vi "Temperature Warnings.vi"(8 "错误输入":cluster{"状态":bool, "代码":i32, "源":string}, 9 "最低温度":dbl, 10 "最高温度":dbl, 11 "当前温度":dbl) -> (0 "错误输出":cluster{"状态":bool, "代码":i32, "源":string}, 2 "警告文本":string="无警告", 3 "警告？":bool)   [LabVIEW 2012]
doc: "该练习将为子VI创建图标和连线板，然后在调用VI中测试调用子VI。"
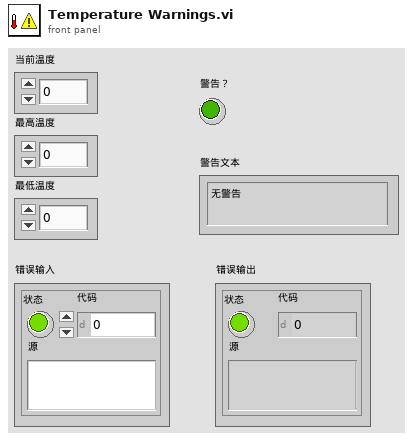
[diagram p1: front panel]
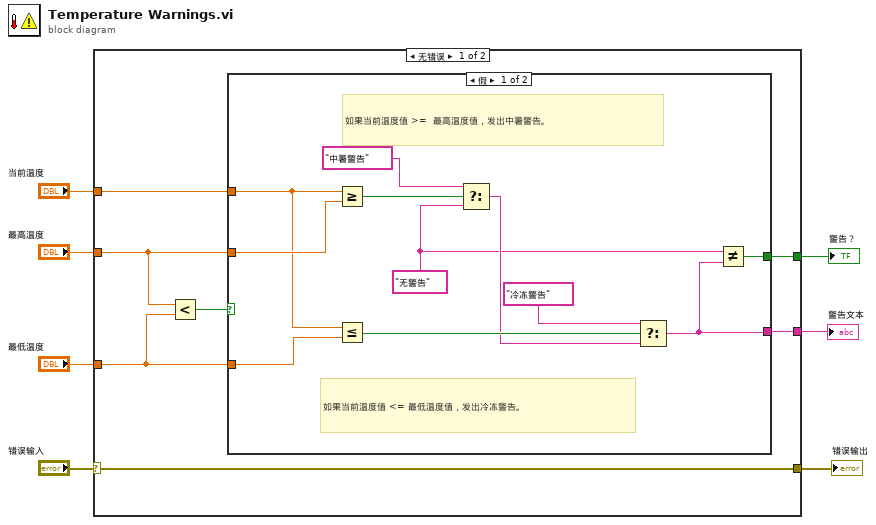
[diagram p0: block diagram]
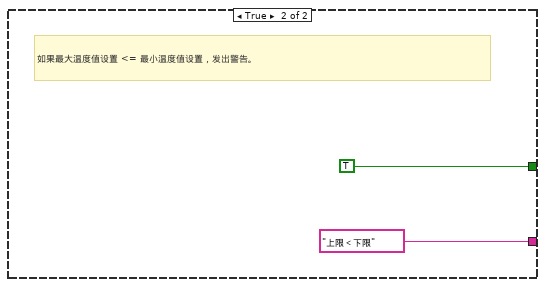
[diagram p2: hidden frame]
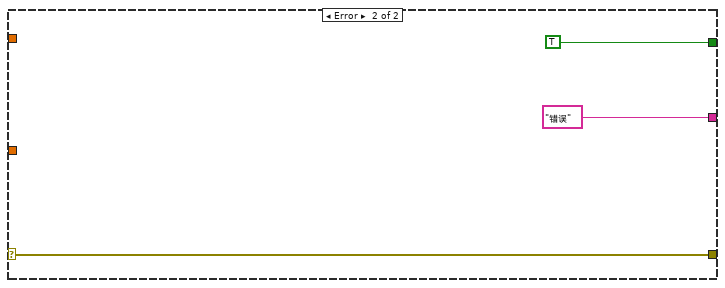
[diagram p3: hidden frame]
diagram:
  n1 = case shown="无错误" "错误输入" {
    selector: "错误输入" -> [w12 w30]
    tunnel: [w14 "错误" ("f")] -> w1
    tunnel: [w13 TRUE] -> w2
    tunnel: [w12 w30] -> w6
    tunnel: "最低温度" -> [w9 _]
    tunnel: "当前温度" -> [w11 _]
    tunnel: "最高温度" -> [w10 _]
    frame No Error {
      n2 = Less? ("小于？")(x=w10, y=w9) -> (x < y?=w8:bool)
      n3 = case shown="假" w8 {
        tunnel: [w15 "上限＜下限" ("f")] -> w14
        tunnel: [w25 TRUE] -> w13
        tunnel: w10 -> [w24 _]
        tunnel: w9 -> [w21 _]
        tunnel: w11 -> [w17 _]
        frame False {
          w16 = "无警告" ("f")
          # "如果当前温度值 >=  最高温度值，发出中暑警告。"
          # "如果当前温度值 <= 最低温度值，发出冷冻警告。"
          n4 = Greater Or Equal? ("大于等于？")(x=w17, y=w24) -> (x >= y?=w23:bool)
          n5 = Less Or Equal? ("小于等于？")(x=w17, y=w21) -> (x <= y?=w19:bool)
          n6 = Select ("选择")(t="中暑警告", s=w23, f=w16) -> (s? t:f=w18:string)
          n7 = Select ("选择")(t="冷冻警告", s=w19, f=w18) -> (s? t:f=w15:string)
          n8 = Not Equal? ("不等于？")(x=w16, y=w15) -> (x != y?=w25:bool)
        }
        frame True {
          # "如果最大温度值设置 <= 最小温度值设置，发出警告。"
        }
      }
    }
    frame Error {
    }
  }
  "错误输出" <- w6
  "警告？" <- w2
  "警告文本" <- w1
